vi "BallPlacementPasserRole.vi"(7 "first call":bool, 8 "error in (no error)":errorcluster, 9 "Tactic index in":i32, 10 "Game in":refnum<class "Game.lvclass">, 11 "BallPlacementPasserRole in":refnum<class "BallPlacementPasserRole.lvclass">) -> (0 "error out":errorcluster, 1 "tactic index out":i32, 2 "Robot out":refnum<class "Robot.lvclass">, 3 "BallPlacementPasserRole out":refnum<class "BallPlacementPasserRole.lvclass">)   [LabVIEW 2021, in "BallPlacementPasserRole.lvclass"]
uses:
  BallPlacementPasserRole.lvclass
  D:/RoboIme/horie/SSL_AI/Role_class/Role.lvclass
  Game_class/Game.lvclass
  Robot_class/Robot.lvclass
  Role_class/Role.lvclass/Role.ctl
  BallPlacementPasserRole.lvclass/BallPlacementPasserRole.ctl
  Tacticbook_class/Tacticbook.lvclass/Tacticbook.ctl
  GoToBallPlacementAllyTactic_class/GoToBallPlacementAllyTactic.lvclass/GoToBallPlacementAllyTactic.ctl
  KickToBestRobotTactic_class/KickToBestRobotTactic.lvclass/KickToBestRobotTactic.ctl
  BallPlacementEnemyTactic_class/BallPlacementEnemyTactic.lvclass/BallPlacementEnemyTactic.ctl
  Tacticbook_class/Read GoToBallPlacementAllyTactic.vi
  GoToBallPlacementAllyTactic_class/Read States.vi
  Tacticbook_class/Write GoToBallPlacementAllyTactic.vi
  KickToBestRobotTactic_class/Read States.vi
  BallPlacementEnemyTactic_class/Read States.vi
  Role_class/Read Tacticbook.vi
  Read number_of_tactics.vi
  Role_class/Read RobotRef.vi
  Role_class/Write Tacticbook.vi
  Role_class/Write tactic_index.vi
  Tacticbook_class/Tacticbook.lvclass
  GoToBallPlacementAllyTactic_class/GoToBallPlacementAllyTactic.lvclass
  KickToBestRobotTactic_class/KickToBestRobotTactic.lvclass
  BallPlacementEnemyTactic_class/BallPlacementEnemyTactic.lvclass
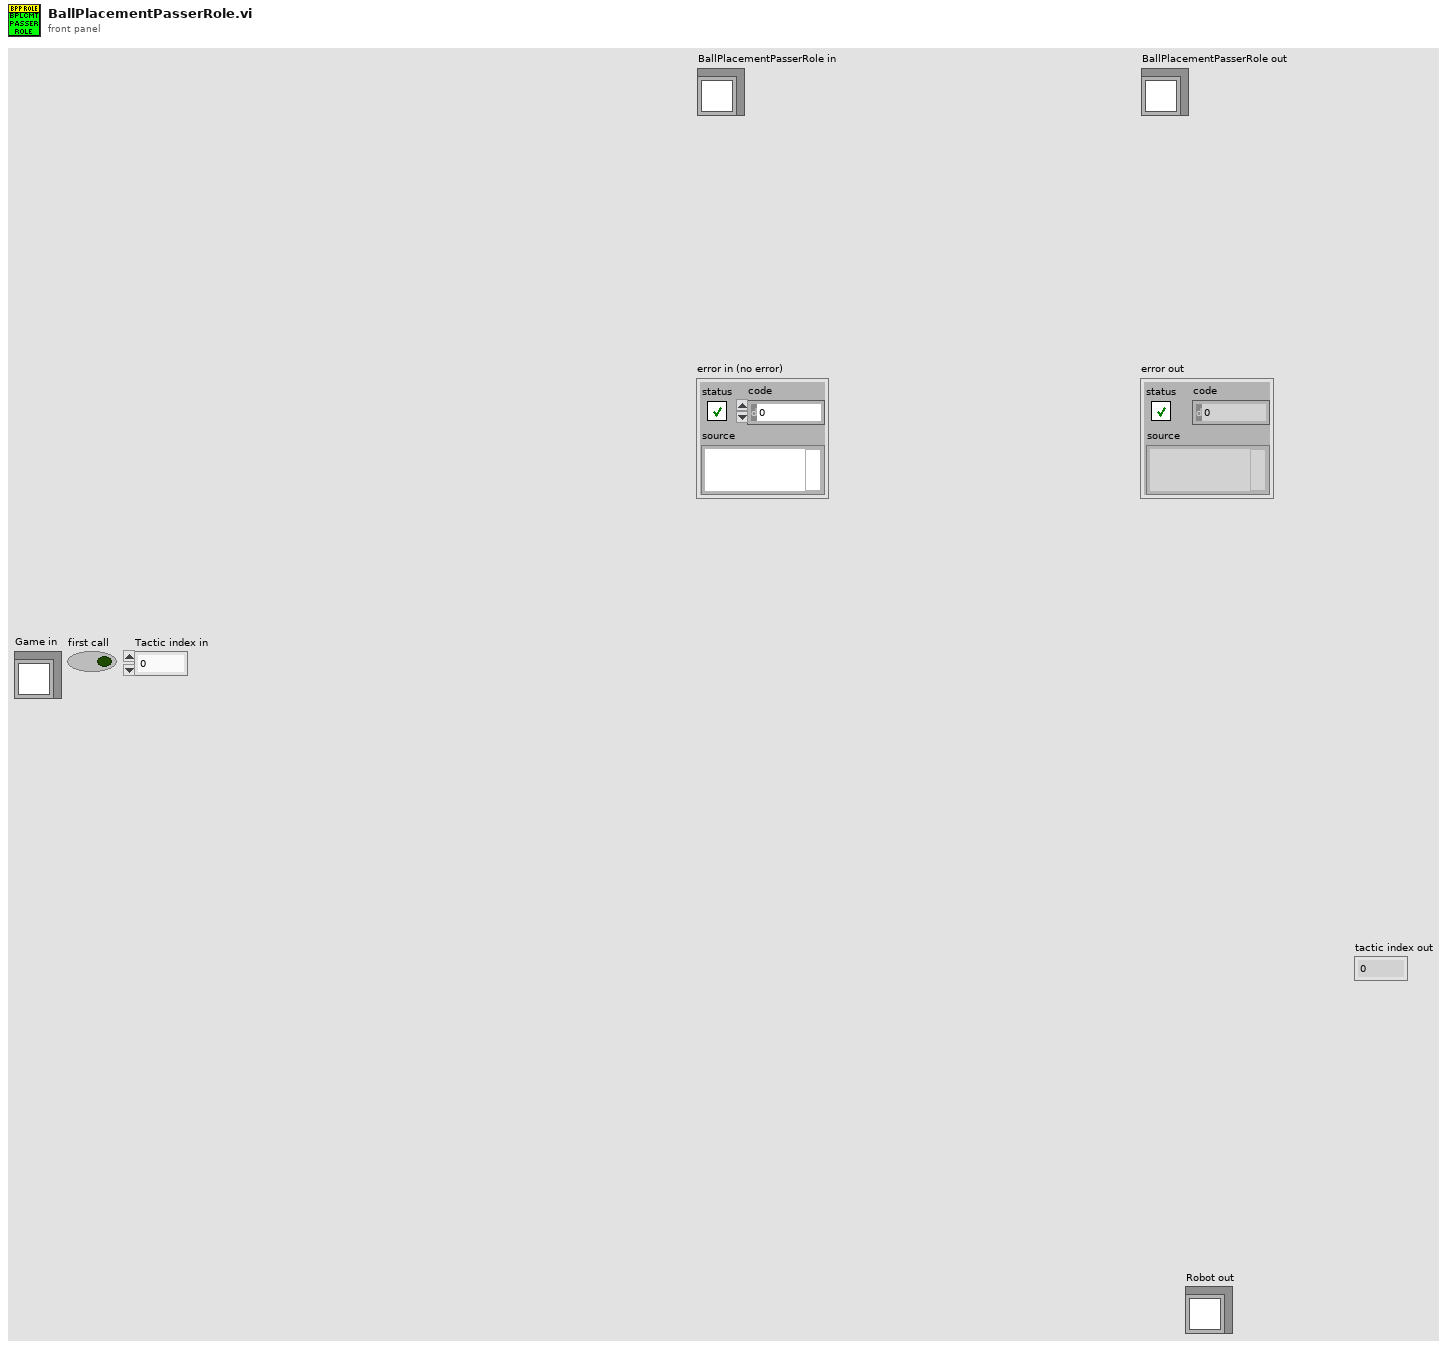
[diagram p1: front panel]
types:
  T1 = typedef "StatesGoToBallPlacementAllyTactic.ctl" = enum16{"GoToNearBall", "GoToBall", "PrepareToPositionBall", "Exit"}
  T2 = typedef "KickToBestRobotTactic.lvclass/KickTOBestRobotTacticStatesEnum.ctl" = enum16{"Pass", "Exit"}
  T3 = typedef "BallPlacementEnemyTactic.lvclass/StatesBallPlacementEnemyTactic.ctl" = enum16{"MoveFromInterference", "Halt", "Exit"}
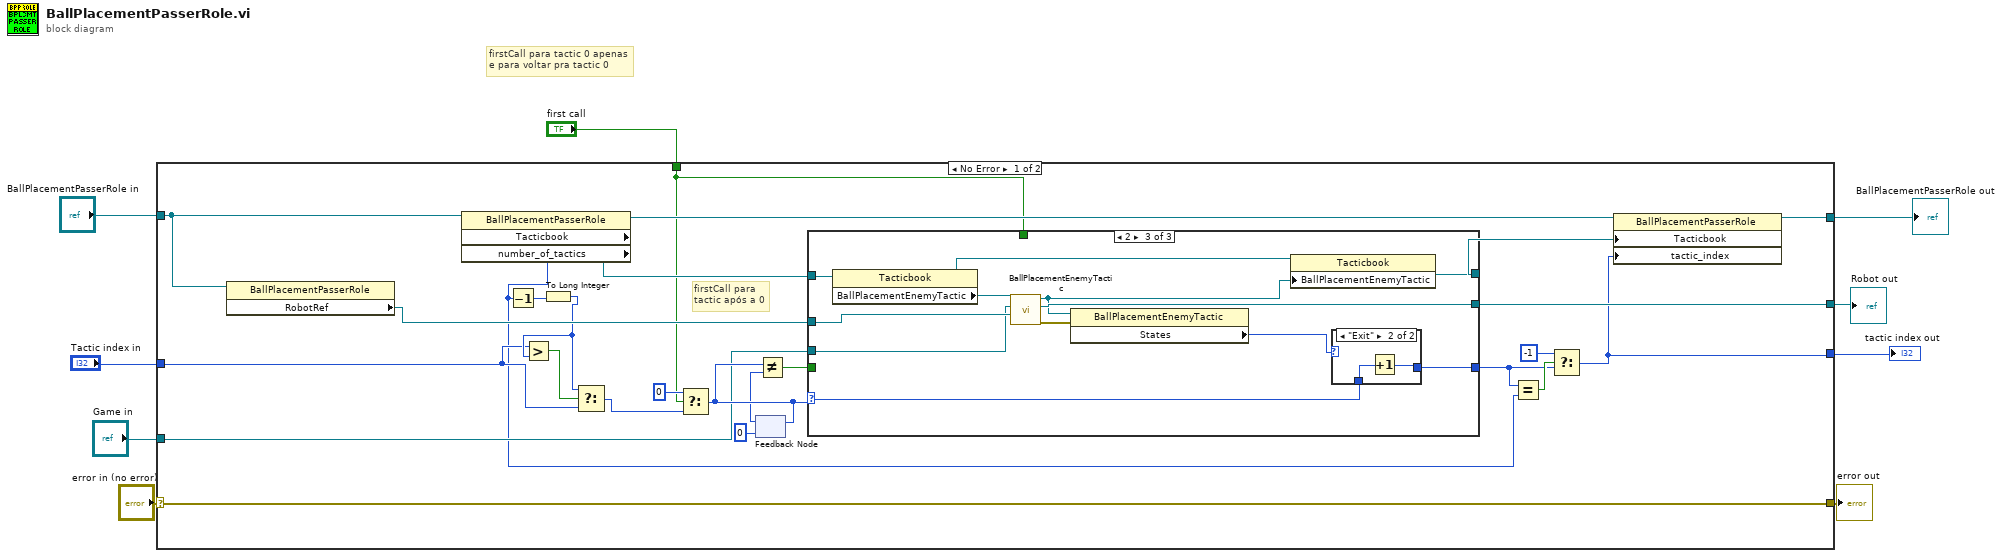
[diagram p0: block diagram]
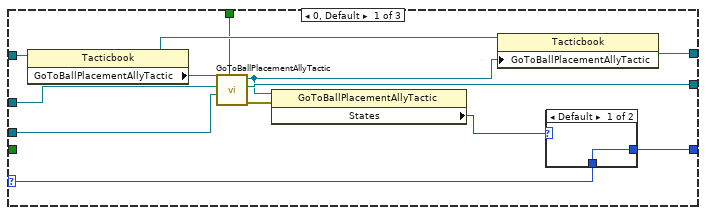
[diagram p2: hidden frame]
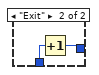
[diagram p3: hidden frame]
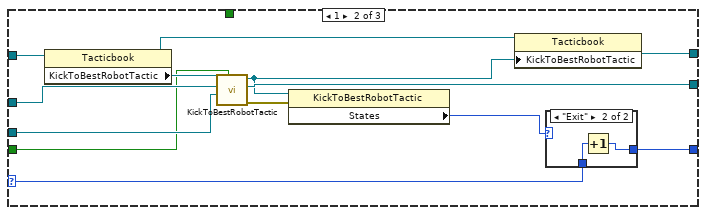
[diagram p4: hidden frame]
diagram:
  # "firstCall para tactic 0 apenas\ne para voltar pra tactic 0"
  n1 = case shown="No Error" "error in (no error)" {
    selector: "error in (no error)" -> [w34 w83]
    tunnel: [w34 w83] -> w8
    tunnel: [w17 w82] -> w6
    tunnel: "BallPlacementPasserRole in" -> [w20 w82]
    tunnel: "Tactic index in" -> [w19 _]
    tunnel: "Game in" -> [w18 _]
    tunnel: "first call" -> [w16 _]
    tunnel: [w10 _] -> w2
    tunnel: [w15 _] -> w1
    frame No Error {
      # "firstCall para\ntactic após a 0"
      n2 = property class="BallPlacementPasserRole"(reference=w20) -> ("RobotRef"=w33:refnum<class "Robot.lvclass">)  [unwired: 1 in, 2 out]
      n3 = property class="BallPlacementPasserRole"(reference=w20) -> (reference out=w32:refnum<class "BallPlacementPasserRole.lvclass">, "Tacticbook"=w31:refnum<class "Tacticbook.lvclass">, "number_of_tactics"=w11:i32)  [unwired: 1 in, 1 out]
      n4 = Decrement(x=w11) -> (x-1=w28:i32)
      n5 = To Long Integer(number=w28) -> (32bit integer=w27:i32)
      n6 = Greater?(x=w19, y=w27) -> (0:w29:bool)
      n7 = Select(t=w27, s=w29, f=w19) -> (s? t:f=w26:i32)
      n8 = Select(t=0, s=w16, f=w26) -> (s? t:f=w24:i32)
      n9 = feedback #1(0 ("Tactic index in")) -> (w23:i32)
      n10 = feedback-in #1(w24) -> ()
      n11 = Not Equal?(x=w24, y=w23) -> (x != y?=w21:bool)
      n12 = case shown="2" w24 {
        selector: w24 -> [w36 w52 w68]
        tunnel: [w44 w60 w75] -> w12
        tunnel: w31 -> [w47 w63 w78]
        tunnel: w33 -> [w40 w57 w72]
        tunnel: [w45 w61 w76] -> w30
        tunnel: w18 -> [w39 w56 w71]
        tunnel: w16 -> [w42 _ _]
        tunnel: [w38 w55 w70] -> w15
        tunnel: w21 -> [_ w53 _]
        frame 0, Default {
          n13 = property class="Tacticbook"(reference=w47) -> (reference out=w46:refnum<class "Tacticbook.lvclass">, "GoToBallPlacementAllyTactic"=w41:refnum<class "GoToBallPlacementAllyTactic.lvclass">)  [unwired: 1 in, 1 out]
          n14 = call "GoToBallPlacementAllyTactic.vi"("firstCall"=w42, "Game in"=w39, "Robot"=w40, "GoToBallPlacementAllyTactic in"=w41) -> ("error out"=w43:errorcluster, "Robot out"=w38:refnum<class "Robot.lvclass">, "GoToBallPlacementAllyTactic out"=w37:refnum<class "GoToBallPlacementAllyTactic.lvclass">)  [unwired: 5 in]
          n15 = property class="GoToBallPlacementAllyTactic"(reference=w37, error in=w43) -> ("States"=w35:T1)  [unwired: 2 out]
          n16 = property class="Tacticbook"(reference=w46, "GoToBallPlacementAllyTactic"=w37) -> (reference out=w45:refnum<class "Tacticbook.lvclass">)  [unwired: 1 in, 1 out]
          n17 = case shown="Default" w35 {
            tunnel: [w48 w49] -> w44
            tunnel: w36 -> [w48 w50]
            frame Default {
            }
            frame "Exit" {
              n18 = Increment(x=w50) -> (x+1=w49:i32)
            }
          }
        }
        frame 1 {
          n19 = property class="Tacticbook"(reference=w63) -> (reference out=w62:refnum<class "Tacticbook.lvclass">, "KickToBestRobotTactic"=w58:refnum<class "KickToBestRobotTactic.lvclass">)  [unwired: 1 in, 1 out]
          n20 = call-dynamic "KickToBestRobotTactic.vi"("first call"=w53, "Game in"=w56, "Robot"=w57, "KickToBestRobotTactic in"=w58) -> ("error out"=w59:errorcluster, "Robot out"=w55:refnum<class "Robot.lvclass">, "KickToBestRobotTactic out"=w54:refnum<class "KickToBestRobotTactic.lvclass">)  [unwired: 4 in, 1 out]
          n21 = property class="KickToBestRobotTactic"(reference=w54, error in=w59) -> ("States"=w51:T2)  [unwired: 2 out]
          n22 = property class="Tacticbook"(reference=w62, "KickToBestRobotTactic"=w54) -> (reference out=w61:refnum<class "Tacticbook.lvclass">)  [unwired: 1 in, 1 out]
          n23 = case shown="\"Exit\"" w51 {
            tunnel: [w64 w65] -> w60
            tunnel: w52 -> [w64 w66]
            frame Default {
            }
            frame "Exit" {
              n24 = Increment(x=w66) -> (x+1=w65:i32)
            }
          }
        }
        frame 2 {
          n25 = property class="Tacticbook"(reference=w78) -> (reference out=w77:refnum<class "Tacticbook.lvclass">, "BallPlacementEnemyTactic"=w73:refnum<class "BallPlacementEnemyTactic.lvclass">)  [unwired: 1 in, 1 out]
          n26 = call "BallPlacementEnemyTactic.vi"("Robot"=w72, "Game"=w71, "BallPlacementEnemyTactic in"=w73) -> ("error out"=w74:errorcluster, "Robot out"=w70:refnum<class "Robot.lvclass">, "BallPlacementEnemyTactic out"=w69:refnum<class "BallPlacementEnemyTactic.lvclass">)  [unwired: 6 in]
          n27 = property class="BallPlacementEnemyTactic"(reference=w69, error in=w74) -> ("States"=w67:T3)  [unwired: 2 out]
          n28 = property class="Tacticbook"(reference=w77, "BallPlacementEnemyTactic"=w69) -> (reference out=w76:refnum<class "Tacticbook.lvclass">)  [unwired: 1 in, 1 out]
          n29 = case shown="\"Exit\"" w67 {
            tunnel: [w79 w81] -> w75
            tunnel: w68 -> [w79 w80]
            frame Default {
            }
            frame "Exit" {
              n30 = Increment(x=w80) -> (x+1=w81:i32)
            }
          }
        }
      }
      n31 = Equal?(x=w12, y=w11) -> (x = y?=w14:bool)
      n32 = Select(t=-1, s=w14, f=w12) -> (s? t:f=w10:i32)
      n33 = property class="BallPlacementPasserRole"(reference=w32, "Tacticbook"=w30, "tactic_index"=w10) -> (reference out=w17:refnum<class "BallPlacementPasserRole.lvclass">)  [unwired: 1 in, 1 out]
    }
    frame Error {
    }
  }
  "error out" <- w8
  "BallPlacementPasserRole out" <- w6
  "Robot out" <- w1
  "tactic index out" <- w2
